vi "ADI_IMU_ADIS16448_Open.vi"(8 "error in 2":errorcluster, 9 "Calibrate On Open 2":bool=TRUE, 10 "AHRS Algorithm 2":enum16{"Complementary", "Madgwick"}(ring), 11 "Yaw Axis 2":enum16{"X", "Y", "Z"}(ring)=enum."Z") -> (0 "error out 2":errorcluster, 1 "error?":bool, 3 "ADI IMU DevRef Out 2":T1={"DevStatus"={"status"=FALSE, "code"=0, "source"=""}, "Handle"=0, "SPI Bus"=enum."SPI On-Board, CS0", "Device Found"=FALSE, "Device Ready"=FALSE, "Yaw Axis"=enum."Z", "AHRS Algorithm"=enum."Complementary", "Serial"=0, "Lot ID 2"=0, "Lot ID 1"=0, "Bytes Per Sample"=0, "Calibrate On Open?"=FALSE})   [LabVIEW 2018, in "ADIS16448_IMU.lvlib"]
doc: "Initiates communication between an Analog Devices MXP IMU and the RoboRIO."
uses:
  ADIS16448_IMU.lvlib
  ADI_IMU_ADIS16448_IMUDevRef.ctl
  <vilib>/Rock Robotics/SystemInterfaces/spilib/spi_bus.ctl
  <vilib>/Rock Robotics/WPI/SPI/WPI_SPIMode.ctl
  <vilib>/Rock Robotics/SystemInterfaces/DIO/FPGA_DIOChannel.ctl
  ADI_IMU_ADIS16448_Registers.ctl
  <vilib>/Rock Robotics/SystemInterfaces/NetworkCommunication/NetComm_UsageReport_ResourceType.ctl
  <vilib>/Utility/error.llb/DialogType.ctl
  <vilib>/Rock Robotics/WPI/Counter/WPI_CounterDigitalInputToDigitalSource.vi
  ADI_IMU_ADIS16448_Loop.vi
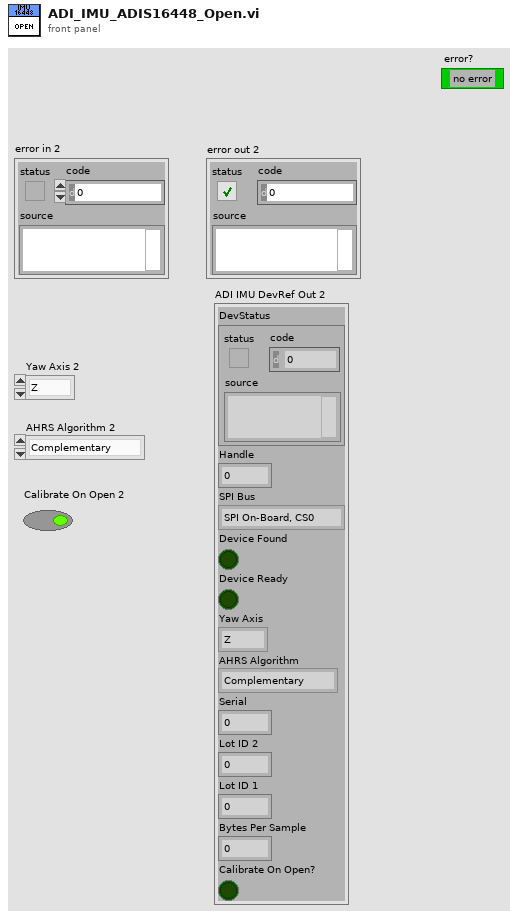
[diagram p1: front panel]
types:
  T1 = typedef "ADIS16448_IMU.lvlib/ADI_IMU_ADIS16448_IMUDevRef.ctl" = cluster{"DevStatus":errorcluster, "Handle":i32, "SPI Bus":T2, "Device Found":bool, "Device Ready":bool, "Yaw Axis":enum16{"X", "Y", "Z"}, "AHRS Algorithm":enum16{"Complementary", "Madgwick"}, "Serial":u16, "Lot ID 2":u16, "Lot ID 1":u16, "Bytes Per Sample":u16, "Calibrate On Open?":bool}
  T2 = typedef "spi_bus.ctl" = enum16{"SPI On-Board, CS0", "SPI On-Board, CS1", "SPI On-Board, CS2", "SPI On-Board, CS3", "SPI MXP", "Invalid"}
  T3 = typedef "FPGA_DIOChannel.ctl" = enum8{"DIO 0", "DIO 1", "DIO 2", "DIO 3", "DIO 4", "DIO 5", "DIO 6", "DIO 7", "DIO 8", "DIO 9", "DIO MXP 0", "DIO MXP 1", "DIO MXP 2", "DIO MXP 3", "DIO MXP 4", "DIO MXP 5", "DIO MXP 6", "DIO MXP 7", "DIO MXP 8", "DIO MXP 9", "DIO MXP 10", "DIO MXP 11", "DIO MXP 12", "DIO MXP 13", "DIO MXP 14", "DIO MXP 15", "SPI Port CS1", "SPI Port CS2", "SPI Port CS3", "SPI Port MISO", "SPI Port MOSI", "Invalid"}
  T4 = typedef "WPI_SPIMode.ctl" = enum16{"Mode 0 (Clk Idle Low,Sample on Leading)", "Mode 1 (Clk Idle Low,Sample on Trailing)", "Mode 2 (Clk Idle High,Sample on Leading)", "Mode 3 (Clk Idle High,Sample on Trailing)"}
  T5 = typedef "NetComm_UsageReport_ResourceType.ctl" = enum8{"Controller", "Module", "Language", "CANPlugin", "Accelerometer", "ADXL345", "AnalogChannel", "AnalogTrigger", "AnalogTriggerOutput", "CANJaguar", "Compressor", "Counter", "Dashboard", "DigitalInput", "DigitalOutput", "DriverStationCIO", "DriverStationEIO", "DriverStationLCD", "Encoder", "GearTooth", "Gyro", "I2C", "Framework", "Jaguar", "Joystick", "Kinect", "KinectStick", "PIDController", "Preferences", "PWM", "Relay", "RobotDrive", "SerialPort", "Servo", "Solenoid", "SPI", "Task", "Ultrasonic", "Victor", "Button", "Command", "AxisCamera", "PCVideoServer", "SmartDashboard", "Talon", "HiTechnicColorSensor", "HiTechnicAccel", "HiTechnicCompass", "SRF08", "AnalogOutput", "Victor SP", "Talon SRX", "CAN Talon SRX", "ADXL362 Accel", "ADXRS450 Gyro", "Rev SPARK", "Mindsensors SD540", "Digital Filter", "ADIS16448", "PDP", "PCM", "PigeonIMU", "Nidec Brushless", "CTRE CANifier", "CTRE Future 0", "CTRE Future 1", "CTRE Future 2", "CTRE Future 3", "CTRE Future 4", "CTRE Future 5", "CTRE Future 6", "Linear Filter", "Xbox Controller", "USB Camera", "NavX", "Pixy", "Pixy2", "ScanseSweep", "Shuffleboard", "CAN", "Digilent DMC60", "PWM Victor SPX", "Rev SPARK MAX PWM", "Rev SPARK MAX CAN", "ADIS16470"}
  T6 = typedef "ADIS16448_IMU.lvlib/ADI_IMU_ADIS16448_Registers.ctl" = u8
  T7 = typedef "WPI_DigitalOutputDevRef.ctl" = cluster{"DIO Channel":T3, "DevStatus":errorcluster}
  T8 = typedef "WPI_DigitalInputDevRef.ctl" = cluster{"DevStatus":errorcluster, "DIO Channel":T3}
  T9 = typedef "WPI_SPIDevRef.ctl" = cluster{"DevStatus":errorcluster, "Handle":i32, "SPI Bus":T2}
  T10 = typedef "FPGA_CounterEncoderSourceConvertionLVSourceType.ctl" = cluster{"DevStatus":errorcluster, "AnalogTriggerMode?":bool, "DigitalMode":cluster{"DIO Channel":T11}, "AnalogTriggerMode":cluster{"AnalogTriggerIndex":T12, "OutputType":T13}}
  T11 = typedef "FPGA_DIODigitalSourceChannel.ctl" = enum8{"DIO 0", "DIO 1", "DIO 2", "DIO 3", "DIO 4", "DIO 5", "DIO 6", "DIO 7", "DIO 8", "DIO 9", "DIO MXP 0", "DIO MXP 1", "DIO MXP 2", "DIO MXP 3", "DIO MXP 4", "DIO MXP 5", "DIO MXP 6", "DIO MXP 7", "DIO MXP 8", "DIO MXP 9", "DIO MXP 10", "DIO MXP 11", "DIO MXP 12", "DIO MXP 13", "DIO MXP 14", "DIO MXP 15", "SPI Port CS1", "SPI Port CS2", "SPI Port CS3", "SPI Port MISO", "SPI Port MOSI", "Disabled"}
  T12 = typedef "FPGA_AnalogTriggerIndex.ctl" = enum8{"Trig 0", "Trig 1", "Trig 2", "Trig 3", "Trig 4", "Trig 5", "Trig 6", "Trig 7", "Invalid"}
  T13 = typedef "FPGA_AnalogTriggerOutType.ctl" = enum16{"InWindow", "TriggerState", "Rising", "Falling"}
  T14 = typedef "DialogType.ctl" = u16
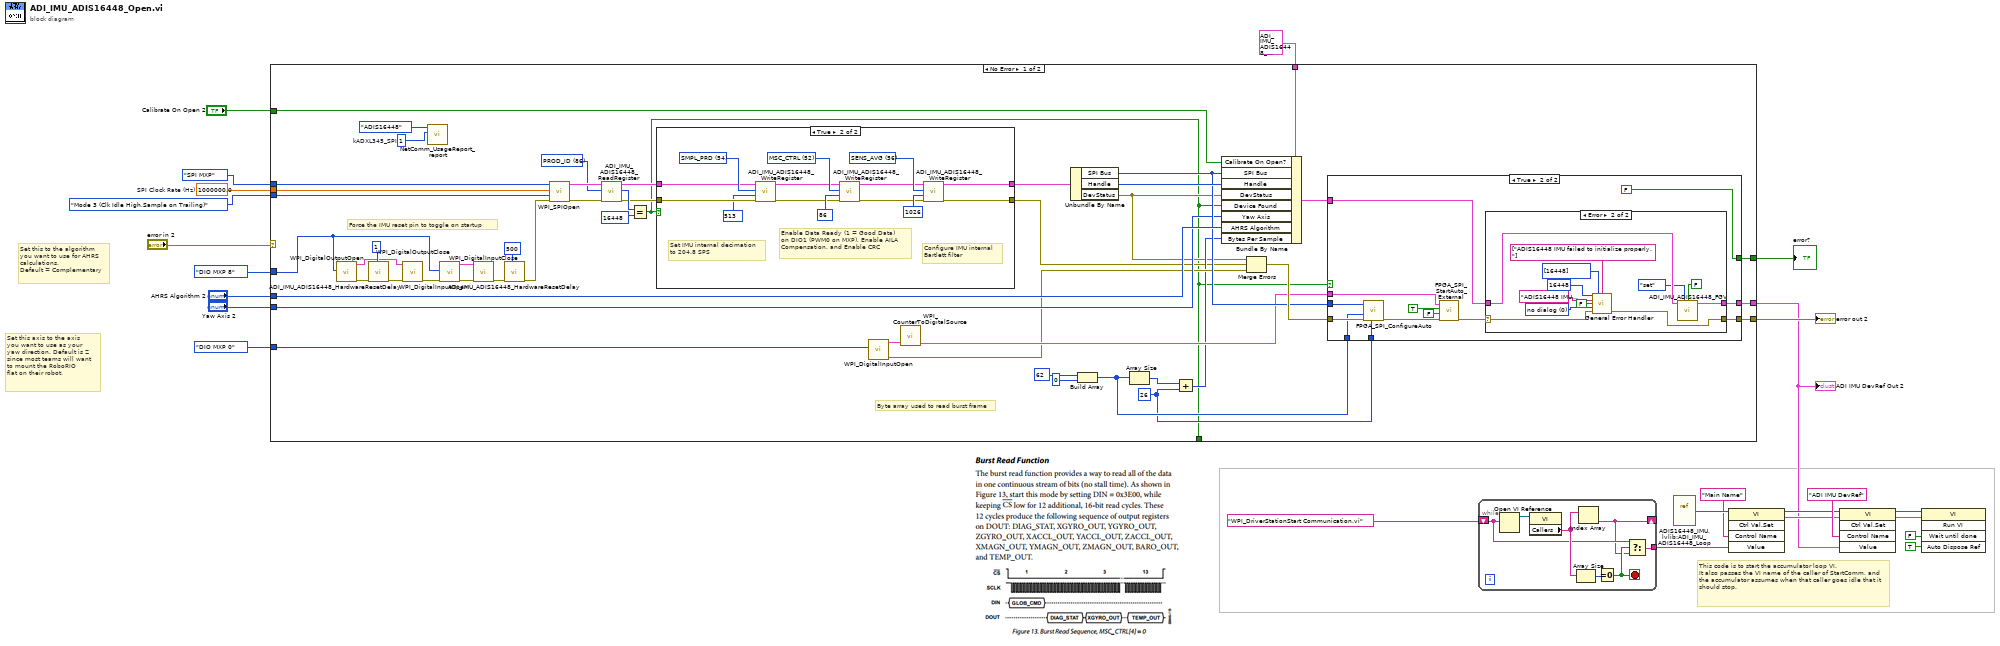
[diagram p0: block diagram]
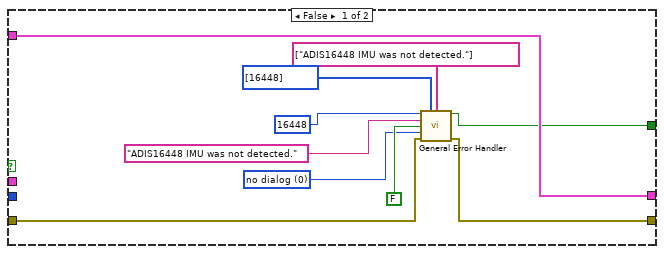
[diagram p2: hidden frame]
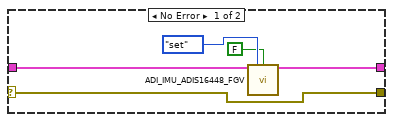
[diagram p3: hidden frame]
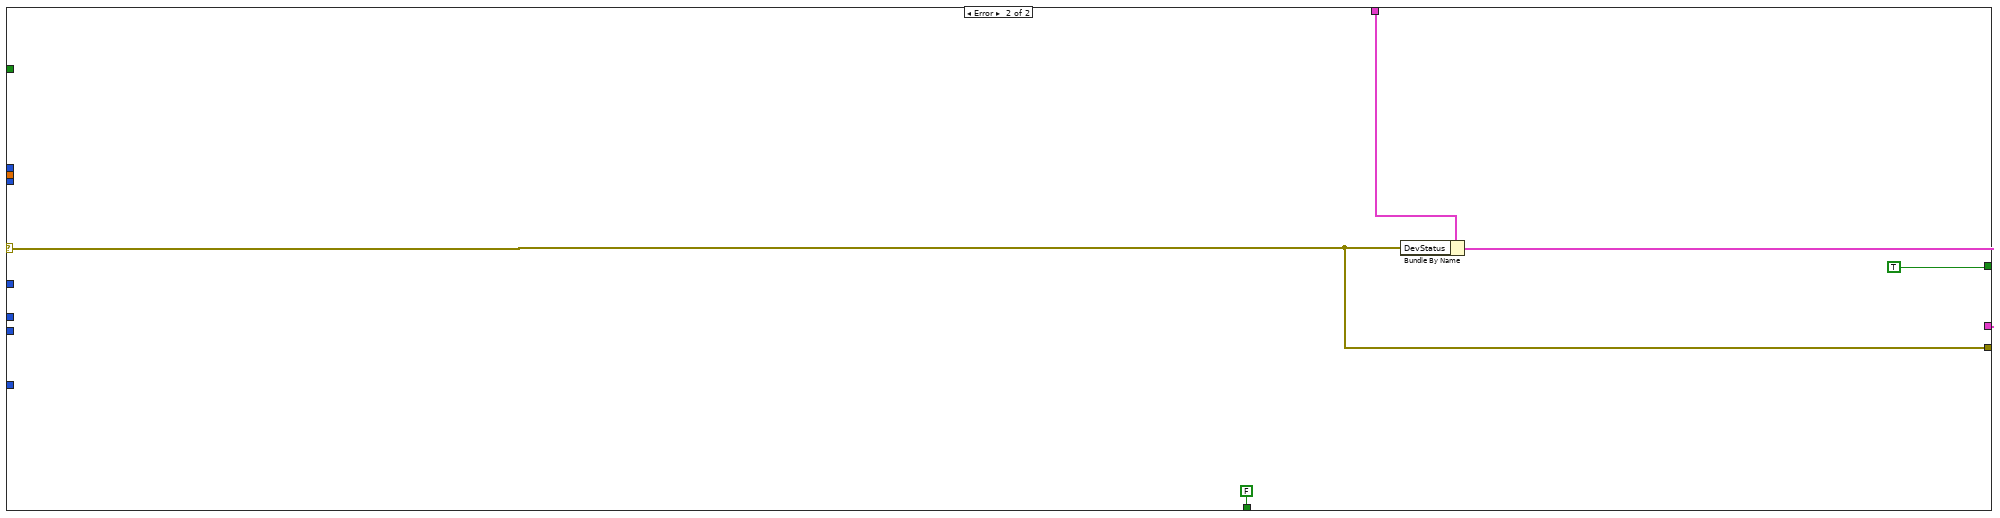
[diagram p5: hidden frame]
diagram:
  w24 = 1000000.0  # SPI Clock Rate (Hz)
  # "This code is to start the accumulator loop VI.\nIt also passes the VI name of the caller of StartComm, and the accumulator assumes when that caller goes idle that it should stop."
  # "Set this to the algorithm\nyou want to use for AHRS\ncalculations. \nDefault = Complementary"
  # "Set this axis to the axis\nyou want to use as your\nyaw direction. Default is Z\nsince most teams will want \nto mount the RoboRIO\nflat on their robot."
  n1 = case shown="No Error" "error in 2" {
    selector: "error in 2" -> [_ w132]
    tunnel: w24 -> [w72 _]
    tunnel: WPI_SPIMode."Mode 3 (Clk Idle High,Sample on Trailing)" ("Mode (3)") -> [w71 _]
    tunnel: spi_bus."SPI MXP" ("SPI Chip Select") -> [w70 _]
    tunnel: FPGA_DIOChannel."DIO MXP 0" ("DIO Channel") -> [w53 _]
    tunnel: "Yaw Axis 2" -> [w50 _]
    tunnel: "AHRS Algorithm 2" -> [w69 _]
    tunnel: FPGA_DIOChannel."DIO MXP 8" ("DIO Channel") -> [w68 _]
    tunnel: "Calibrate On Open 2" -> [w34 _]
    tunnel: T1 {"DevStatus"={"status"=FALSE, "code"=0, "source"=""}, "Handle"=0, "SPI Bus"=enum."SPI On-Board, CS0", "Device Found"=FALSE, "Device Ready"=FALSE, "Yaw Axis"=enum."Z", "AHRS Algorithm"=enum."Complementary", "Serial"=0, "Lot ID 2"=0, "Lot ID 1"=0, "Bytes Per Sample"=0, "Calibrate On Open?"=FALSE} ("SimpleGyroDevRef 2") -> [w49 w133]
    tunnel: [w48 w132] -> w4
    tunnel: [w27 w131] -> w3
    tunnel: [w26 FALSE] -> _
    tunnel: [w25 TRUE] -> w1
    frame No Error {
      w31 = 26 ("dimension size")
      w65 = u8 1  # kADXL345_SPI
      w61 = T6 86 items=["GLOB_CMD"=62, "SEQ_CNT"=58, "SMPL_PRD"=54, "SENS_AVG"=56, "MSC_CTRL"=52, "ERROR_FLAGS"=60, "TEMP"=44, "BARO"=40, "Z_MAG"=36, "Y_MAG"=32, "X_MAG"=28, "Z_ACCEL"=24, "Y_ACCEL"=20, "X_ACCEL"=16, "Z_GYRO"=12, "Y_GYRO"=8, "X_GYRO"=4, "PROD_ID"=86, "LOT_ID2"=84, "LOT_ID1"=82, "SERIAL_NUM"=88] ("ADIS16448 Register")
      # "Byte array used to read burst frame"
      # "Force the IMU reset pin to toggle on startup"
      n2 = call <vilib>:"WPI_DigitalOutputOpen.vi"("DIO Channel"=w68) -> ("error out"=w45:errorcluster, "DigitalOutputDevRef"=w39:T7)  [unwired: 9 in]
      n3 = call "ADI_IMU_ADIS16448_HardwareResetDelay.vi"("Delay (ms)"=u32 1, "error in"=w45) -> ("error out"=w46:errorcluster)  [unwired: 9 in]
      n4 = call <vilib>:"WPI_DigitalOutputClose.vi"("error in (no error)"=w46, "DigitalOutputDevRef"=w39) -> ("error out"=w44:errorcluster)  [unwired: 9 in]
      n5 = call <vilib>:"NetComm_UsageReport_report.vi"("Instance Number"=w65, "Resource Type"=NetComm_UsageReport_ResourceType."ADIS16448") -> ()  [unwired: 10 in]
      n6 = call <vilib>:"WPI_DigitalInputOpen.vi"("error in (no error)"=w44, "DIO Channel"=w68) -> ("error out"=w43:errorcluster, "DigitalInputDevRef"=w42:T8)  [unwired: 8 in]
      n7 = call <vilib>:"WPI_DigitalInputClose.vi"("error in (no error)"=w43, "DigitalInputDevRef"=w42) -> ("error out"=w41:errorcluster)  [unwired: 9 in]
      n8 = call "ADI_IMU_ADIS16448_HardwareResetDelay.vi"("Delay (ms)"=u32 500, "error in"=w41) -> ("error out"=w66:errorcluster)  [unwired: 9 in]
      n9 = call <vilib>:"WPI_SPIOpen.vi"("error in"=w66, "Mode (3)"=w71, "Clock Rate (Hz)"=w72, "SPI Bus"=w70) -> ("error out"=w62:errorcluster, "SPIDevRef"=w63:T9)  [unwired: 6 in]
      n10 = call "ADI_IMU_ADIS16448_ReadRegister.vi"("error in (no error)"=w62, "ADIS16448 Register"=w61, "SPIDevRef in"=w63) -> ("error out"=w57:errorcluster, "Register Value"=w60:u16, "SPIDevRef out"=w58:T9)  [unwired: 6 in]
      n11 = Equal?(x=w60, y=u16 16448) -> (x = y?=w26:bool)
      n12 = case shown="True" w26 {
        tunnel: [w114 w116] -> w56
        tunnel: [w113 w115] -> w29
        tunnel: w58 -> [w114 w119]
        tunnel: w57 -> [w113 w118]
        frame False {
        }
        frame True {
          w124 = T6 56 items=["GLOB_CMD"=62, "SEQ_CNT"=58, "SMPL_PRD"=54, "SENS_AVG"=56, "MSC_CTRL"=52, "ERROR_FLAGS"=60, "TEMP"=44, "BARO"=40, "Z_MAG"=36, "Y_MAG"=32, "X_MAG"=28, "Z_ACCEL"=24, "Y_ACCEL"=20, "X_ACCEL"=16, "Z_GYRO"=12, "Y_GYRO"=8, "X_GYRO"=4, "PROD_ID"=86, "LOT_ID2"=84, "LOT_ID1"=82, "SERIAL_NUM"=88] ("ADIS16448 Register")
          w125 = T6 52 items=["GLOB_CMD"=62, "SEQ_CNT"=58, "SMPL_PRD"=54, "SENS_AVG"=56, "MSC_CTRL"=52, "ERROR_FLAGS"=60, "TEMP"=44, "BARO"=40, "Z_MAG"=36, "Y_MAG"=32, "X_MAG"=28, "Z_ACCEL"=24, "Y_ACCEL"=20, "X_ACCEL"=16, "Z_GYRO"=12, "Y_GYRO"=8, "X_GYRO"=4, "PROD_ID"=86, "LOT_ID2"=84, "LOT_ID1"=82, "SERIAL_NUM"=88] ("ADIS16448 Register")
          w126 = T6 54 items=["GLOB_CMD"=62, "SEQ_CNT"=58, "SMPL_PRD"=54, "SENS_AVG"=56, "MSC_CTRL"=52, "ERROR_FLAGS"=60, "TEMP"=44, "BARO"=40, "Z_MAG"=36, "Y_MAG"=32, "X_MAG"=28, "Z_ACCEL"=24, "Y_ACCEL"=20, "X_ACCEL"=16, "Z_GYRO"=12, "Y_GYRO"=8, "X_GYRO"=4, "PROD_ID"=86, "LOT_ID2"=84, "LOT_ID1"=82, "SERIAL_NUM"=88] ("ADIS16448 Register")
          # "Configure IMU internal\nBartlett filter"
          # "Enable Data Ready (1 = Good Data) \non DIO1 (PWM0 on MXP), Enable AILA\nCompensation, and Enable CRC"
          # "Set IMU internal decimation\nto 204.8 SPS"
          n13 = call "ADI_IMU_ADIS16448_WriteRegister.vi"("error in (no error)"=w118, "Data"=u16 513, "ADIS16448 Register"=w126, "SPIDevRef in"=w119) -> ("error out"=w122:errorcluster, "SPIDevRef out"=w123:T9)  [unwired: 6 in]
          n14 = call "ADI_IMU_ADIS16448_WriteRegister.vi"("error in (no error)"=w122, "Data"=u16 86, "ADIS16448 Register"=w125, "SPIDevRef in"=w123) -> ("error out"=w120:errorcluster, "SPIDevRef out"=w121:T9)  [unwired: 6 in]
          n15 = call "ADI_IMU_ADIS16448_WriteRegister.vi"("error in (no error)"=w120, "Data"=u16 1026, "ADIS16448 Register"=w124, "SPIDevRef in"=w121) -> ("error out"=w115:errorcluster, "SPIDevRef out"=w116:T9)  [unwired: 6 in]
        }
      }
      n16 = call <vilib>:"WPI_DigitalInputOpen.vi"("DIO Channel"=w53) -> ("error out"=w38:errorcluster, "DigitalInputDevRef"=w52:T8)  [unwired: 9 in]
      n17 = call-poly <vilib>:"WPI_CounterToDigitalSource.vi"("DigitalInputDevRef"=w52) -> ("Digital Source"=w51:T10)  [unwired: 6 in]
      n18 = Unbundle By Name(w56) -> ("SPI Bus"=w54:T2, "Handle"=w67:i32, "DevStatus"=w30:errorcluster)
      n19 = Build Array(u8 62 ("hi"), u8 0 ("element")) -> (w35:u8[])
      n20 = Array Size(array=w35) -> (size(s)=w33:i32)
      n21 = Add(x=w33, y=w31) -> (x+y=w32:i32)
      n22 = Bundle By Name(cluster=w49, "Calibrate On Open?"=w34, "SPI Bus"=w54, "Handle"=w67, "DevStatus"=w30, "Device Found"=w26, "Yaw Axis"=w50, "AHRS Algorithm"=w69, "Bytes Per Sample"=w32) -> (w28:T1)
      n23 = Merge Errors(w30, w29, w38) -> (w55:errorcluster)
      n24 = case shown="True" w26 {
        tunnel: w55 -> [w75 w95]
        tunnel: w54 -> [_ w94]
        tunnel: w35 -> [_ w89]
        tunnel: w51 -> [_ w90]
        tunnel: [w76 w86] -> w48
        tunnel: w31 -> [_ w88]
        tunnel: w28 -> [w74 w85]
        tunnel: [w74 w84] -> w27
        tunnel: [w73 FALSE] -> w25
        frame False {
          w79 = T14 0 items=["no dialog", "OK message", "continue or stop message", "OK message + warnings", "continue/stop + warnings"] ("type of dialog (OK msg:1)")
          n25 = call <vilib>:"General Error Handler.vi"("[error code] (0)"=16448, "[user-defined codes]"=i32[] [16448], "[user-defined descriptions]"=string[] ["ADIS16448 IMU was not detected."], "[error source] (\" \")"="ADIS16448 IMU was not detected." ("[error source] (\" \")"), "search ni.com link visible?(T)"=FALSE, "type of dialog (OK msg:1)"=w79, "error in (no error)"=w75) -> ("error?"=w73:bool, "error out"=w76:errorcluster)  [unwired: 4 in, 3 out]
        }
        frame True {
          n26 = call <vilib>:"FPGA_SPI_ConfigureAuto.vi"("SPI Auto Zero Byte Count"=w88, "error in"=w95, "SPI Auto TX Byte Array"=w89, "SPI Bus"=w94) -> ("error out"=w93:errorcluster)  [unwired: 7 in]
          n27 = call <vilib>:"FPGA_SPI_StartAuto_External.vi"("error in (no error)"=w93, "Falling Edge"=FALSE, "Rising Edge"=TRUE, "Source"=w90) -> ("error out"=w87:errorcluster)  [unwired: 7 in]
          n28 = case shown="Error" w87 {
            selector: w87 -> [w96 w106]
            tunnel: w85 -> [w97 w104]
            tunnel: [w96 w101] -> w86
            tunnel: [w98 w105] -> w84
            frame No Error {
              n29 = call "ADI_IMU_ADIS16448_FGV.vi"("ADI IMU DevRef"=w97, "Operation"=enum16{"set", "get", "set reset"}."set", "Sensor Ready?"=FALSE) -> ("ADI IMU DevRef Out"=w98:T1)  [unwired: 6 in, 6 out]
            }
            frame Error {
              w109 = T14 0 items=["no dialog", "OK message", "continue or stop message", "OK message + warnings", "continue/stop + warnings"] ("type of dialog (OK msg:1)")
              n30 = call <vilib>:"General Error Handler.vi"("[error code] (0)"=16448, "[user-defined codes]"=i32[] [16448], "[user-defined descriptions]"=string[] ["ADIS16448 IMU failed to initialize properly."], "[error source] (\" \")"="ADIS16448 IMU failed to initialize properly." ("[error source] (\" \")"), "search ni.com link visible?(T)"=FALSE, "type of dialog (OK msg:1)"=w109, "error in (no error)"=w106) -> ("error out"=w101:errorcluster)  [unwired: 4 in, 4 out]
              n31 = call "ADI_IMU_ADIS16448_FGV.vi"("ADI IMU DevRef"=w104, "Operation"=enum16{"set", "get", "set reset"}."set", "Sensor Ready?"=FALSE) -> ("ADI IMU DevRef Out"=w105:T1)  [unwired: 6 in, 6 out]
            }
          }
        }
      }
    }
    frame Error {
      n32 = Bundle By Name(cluster=w133, "DevStatus"=w132) -> (w131:T1)
    }
  }
  "error out 2" <- w4
  "ADI IMU DevRef Out 2" <- w3
  "error?" <- w1
  n33 = while {
    shift-right: [w135] -> _
    shift-left: "WPI_DriverStationStart Communication.vi" -> [w136]
    tunnel: [w134] -> w8
    stop <- w137 stop-if-true
    n34 = Open VI Reference(vi path=w136) -> (vi reference=w140:refnum<vi>)  [unwired: 1 in, 5 out]
    n35 = property class="VI"(reference=w140) -> ("Callers"=w138:string[])  [unwired: 1 in, 2 out]
    n36 = Array Size(array=w138) -> (size(s)=w139:i32)
    n37 = Index Array(array=w138) -> (element=w135:string)  [unwired: 1 in]
    n38 = Equal To 0?(x=w139) -> (x = 0?=w137:bool)
    n39 = Select(t=w136, s=w137, f=w135) -> (s? t:f=w134:string)
  }
  n40 = vi-ref "ADIS16448_IMU.lvlib:ADI_IMU_ADIS16448_Loop.vi"() -> (w10:refnum<vi>)
  n41 = invoke class="VI" method="Ctrl Val.Set"(reference=w10, "Control Name"="Main Name", "Value"=w8) -> (reference out=w7:refnum<vi>, error out=w12:errorcluster)  [unwired: 2 in, 3 out]
  n42 = invoke class="VI" method="Ctrl Val.Set"(reference=w7, error in=w12, "Control Name"="ADI IMU DevRef", "Value"=w3) -> (reference out=w17:refnum<vi>, error out=w13:errorcluster)  [unwired: 1 in, 3 out]
  n43 = invoke class="VI" method="Run VI"(reference=w17, error in=w13, "Wait until done"=FALSE ("Wait Until Done"), "Auto Dispose Ref"=TRUE ("Auto Dispose Reference")) -> ()  [unwired: 1 in, 5 out]
